vi "Drive_Config.vi"(0 "Left_Power in":dbl, 5 "Right_Power in":dbl, 7 "Motor Mode":enum32{"Coast", "Brake"}(radio)) -> (4 "GPIO_Value":bool[](array[boolean]), 6 "PWM_Value":dbl[](array[numeric]), 8 "GPIO_Channels":u8[](array[numeric])=[4, 7, 8, 11, 12], 15 "PWM Channels":u8[](array[numeric])=[9, 10])   [LabVIEW 2018, in "ArgoBotLib.lvlib"]
uses:
  ArgoBotLib.lvlib
panel:
  in  "PWM Motor":u8[](array[numeric])=[3, 5]
  in  "Motor_GPIO_Value":u8[](array[numeric])=[8, 4, 7, 11, 12]
  out "Right_Back":bool
  out "Right_Forward":bool
  out "Right_Power out":dbl
  out "standby":bool
  out "Left_Power out":dbl
  out "Left_Back":bool
  out "Left_Forward":bool
  # "ArgoBot  Drive Config"
  # "This vi take left and right motor and converts it into a version the motor controller can read"
  # "Inputs"
  # "Tunes"
  # "Test Points"
  # "Outputs"
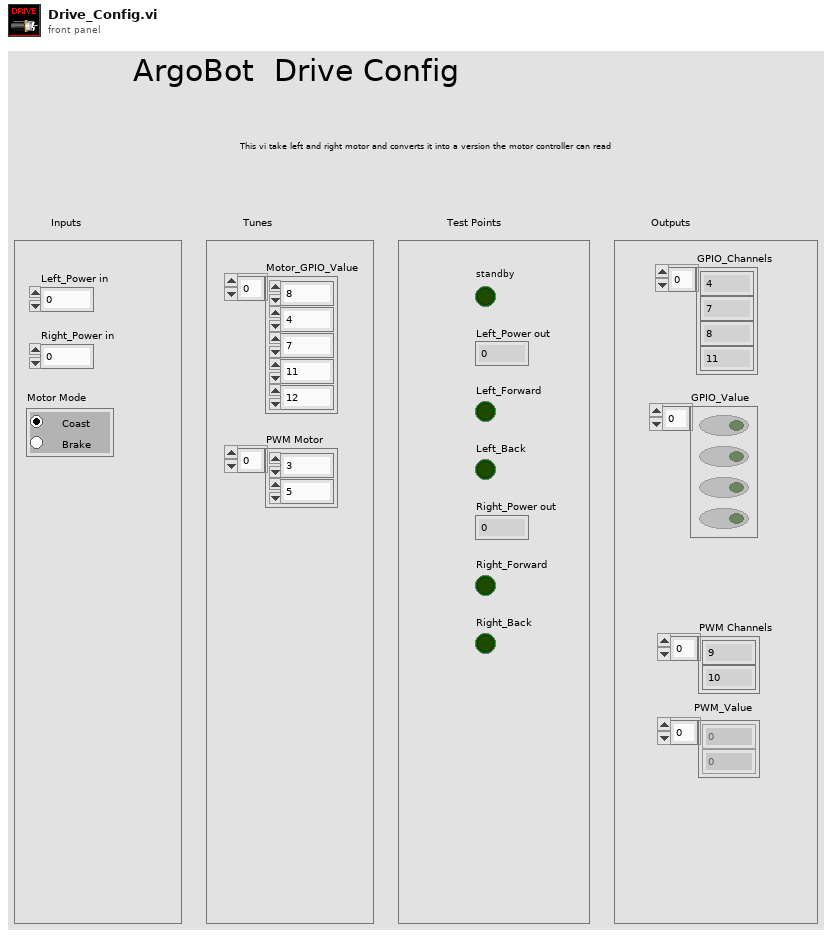
[diagram p1: front panel]
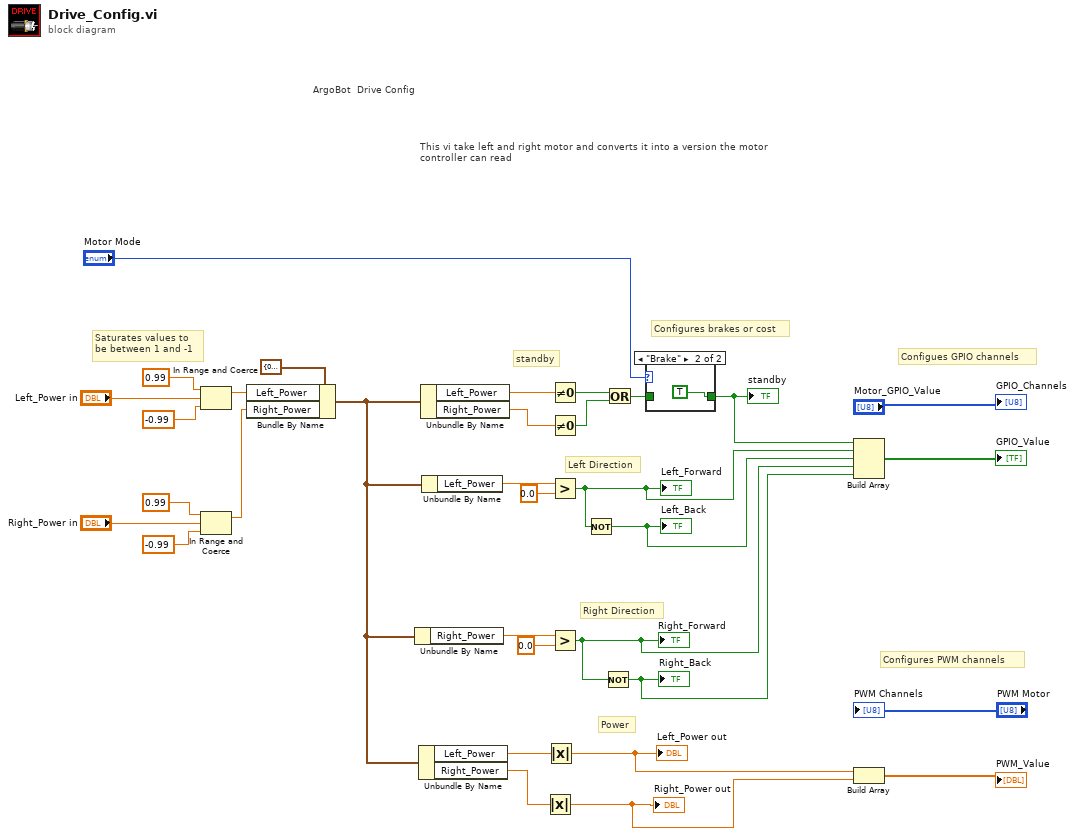
[diagram p0: block diagram]
diagram:
  # "Configures brakes or cost"
  # "Configures PWM channels"
  # "Configues GPIO channels"
  # "Saturates values to \nbe between 1 and -1"
  # "This vi take left and right motor and converts it into a version the motor controller can read"
  # "ArgoBot  Drive Config"
  # "Power"
  # "Right Direction"
  # "Left Direction"
  # "standby"
  n1 = In Range and Coerce(upper limit=0.99, x="Left_Power in", lower limit=-0.99) -> (coerced(x)=w16:dbl)  [unwired: 1 out]
  n2 = In Range and Coerce(upper limit=0.99, x="Right_Power in", lower limit=-0.99) -> (coerced(x)=w17:dbl)  [unwired: 1 out]
  n3 = Bundle By Name(cluster=cluster{"Left_Power":dbl, "Right_Power":dbl} {"Left_Power"=0.0, "Right_Power"=0.0} ("input cluster"), "Left_Power"=w16, "Right_Power"=w17) -> (w27:cluster{"Left_Power":dbl, "Right_Power":dbl})
  n4 = Unbundle By Name(w27) -> ("Right_Power"=w26:dbl)
  n5 = Unbundle By Name(w27) -> ("Left_Power"=w28:dbl, "Right_Power"=w29:dbl)
  n6 = Unbundle By Name(w27) -> ("Left_Power"=w19:dbl, "Right_Power"=w20:dbl)
  n7 = Unbundle By Name(w27) -> ("Left_Power"=w25:dbl)
  n8 = Absolute Value(x=w29) -> (abs(x)=w33:dbl)
  "Right_Power out" <- w33
  n9 = Absolute Value(x=w28) -> (abs(x)=w32:dbl)
  "Left_Power out" <- w32
  n10 = Not Equal To 0?(x=w19) -> (x != 0?=w21:bool)
  n11 = Not Equal To 0?(x=w20) -> (x != 0?=w22:bool)
  n12 = Greater?(x=w25, y=0.0) -> (0:w5:bool)
  "Left_Forward" <- w5
  n13 = Greater?(x=w26, y=0.0) -> (0:w30:bool)
  "Right_Forward" <- w30
  n14 = Not(x=w5) -> (.not. x?=w4:bool)
  "Left_Back" <- w4
  n15 = Not(x=w30) -> (.not. x?=w31:bool)
  "Right_Back" <- w31
  n16 = Or(x=w21, y=w22) -> (x .or. y?=w2:bool)
  n17 = case shown="\"Brake\"" "Motor Mode" {
    tunnel: w2 -> [w34 _]
    tunnel: [w34 TRUE] -> w1
    frame "Coast", Default {
    }
    frame "Brake" {
    }
  }
  "standby" <- w1
  n18 = Build Array(w1, w5, w4, w30, w31) -> (→"GPIO_Value":bool[])
  n19 = Build Array(w32, w33) -> (→"PWM_Value":dbl[])
  "GPIO_Channels" <- "Motor_GPIO_Value"
  "PWM Channels" <- "PWM Motor"
